vi "Create Registry.vi"(8 "Error In":errorcluster) -> (0 "Error Out":errorcluster)   [LabVIEW 2014]
doc: "This subVI creates a registry for registring and control version numbers."
uses:
  <vilib>/Utility/file.llb/Read From Spreadsheet File (string).vi
panel:
  in  "Enum":enum16{"idle", "create", "cancle"}(ring)
  in  "Cancel Button":bool
  in  "Create":bool
  in  "Project Description":string="GFB HIL project setup. Project no. 7152364"
  in  "Delimiter":string=";"
  in  "Project Name":string="Gullfaks B"
  out "ini file path":path
  # "Create Registry"
  # "This application creates a TDMS file that is used to store version numbers\nof all the executables in the HIL setup.\n\nIf the TDMS file has already been created, avoid running this application. Run Update Registry, instead.\n\nTo run this application, you need a database of the components, saved as a CSV file."
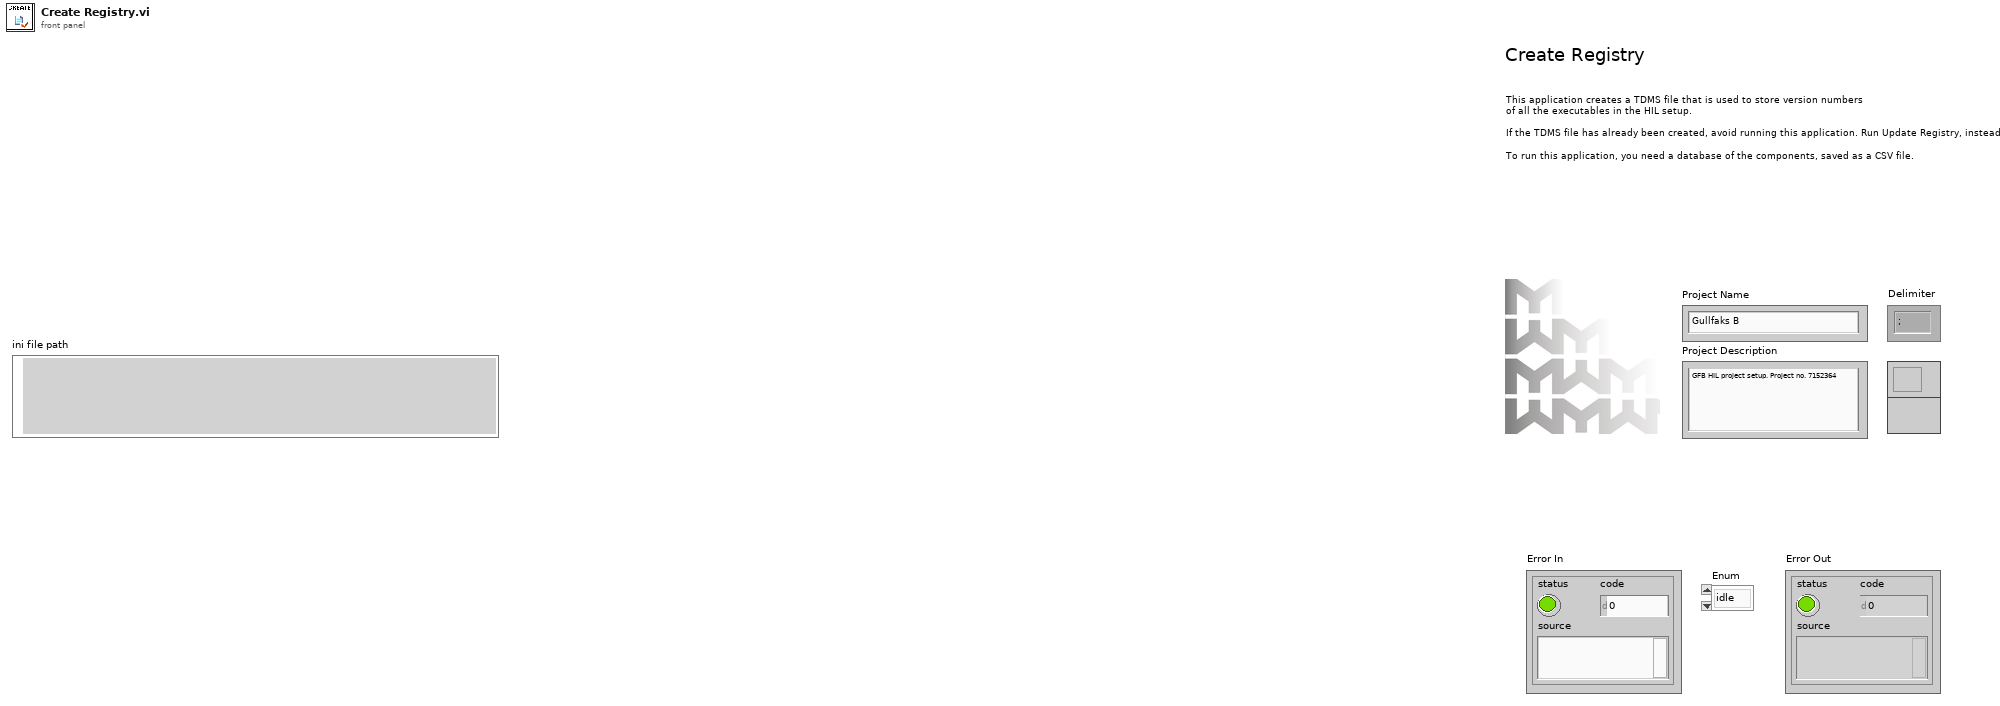
[diagram p1: front panel]
types:
  T1 = cluster{"Folder Path containing version information":path, "File name (including .ini)":path, "Section":string}
  T2 = cluster{"path":path, "This VI":refnum<vi>, "Level of Application":u8}
  T3 = enum16{"open", "open or create", "create or replace", "create", "open (read-only)"}
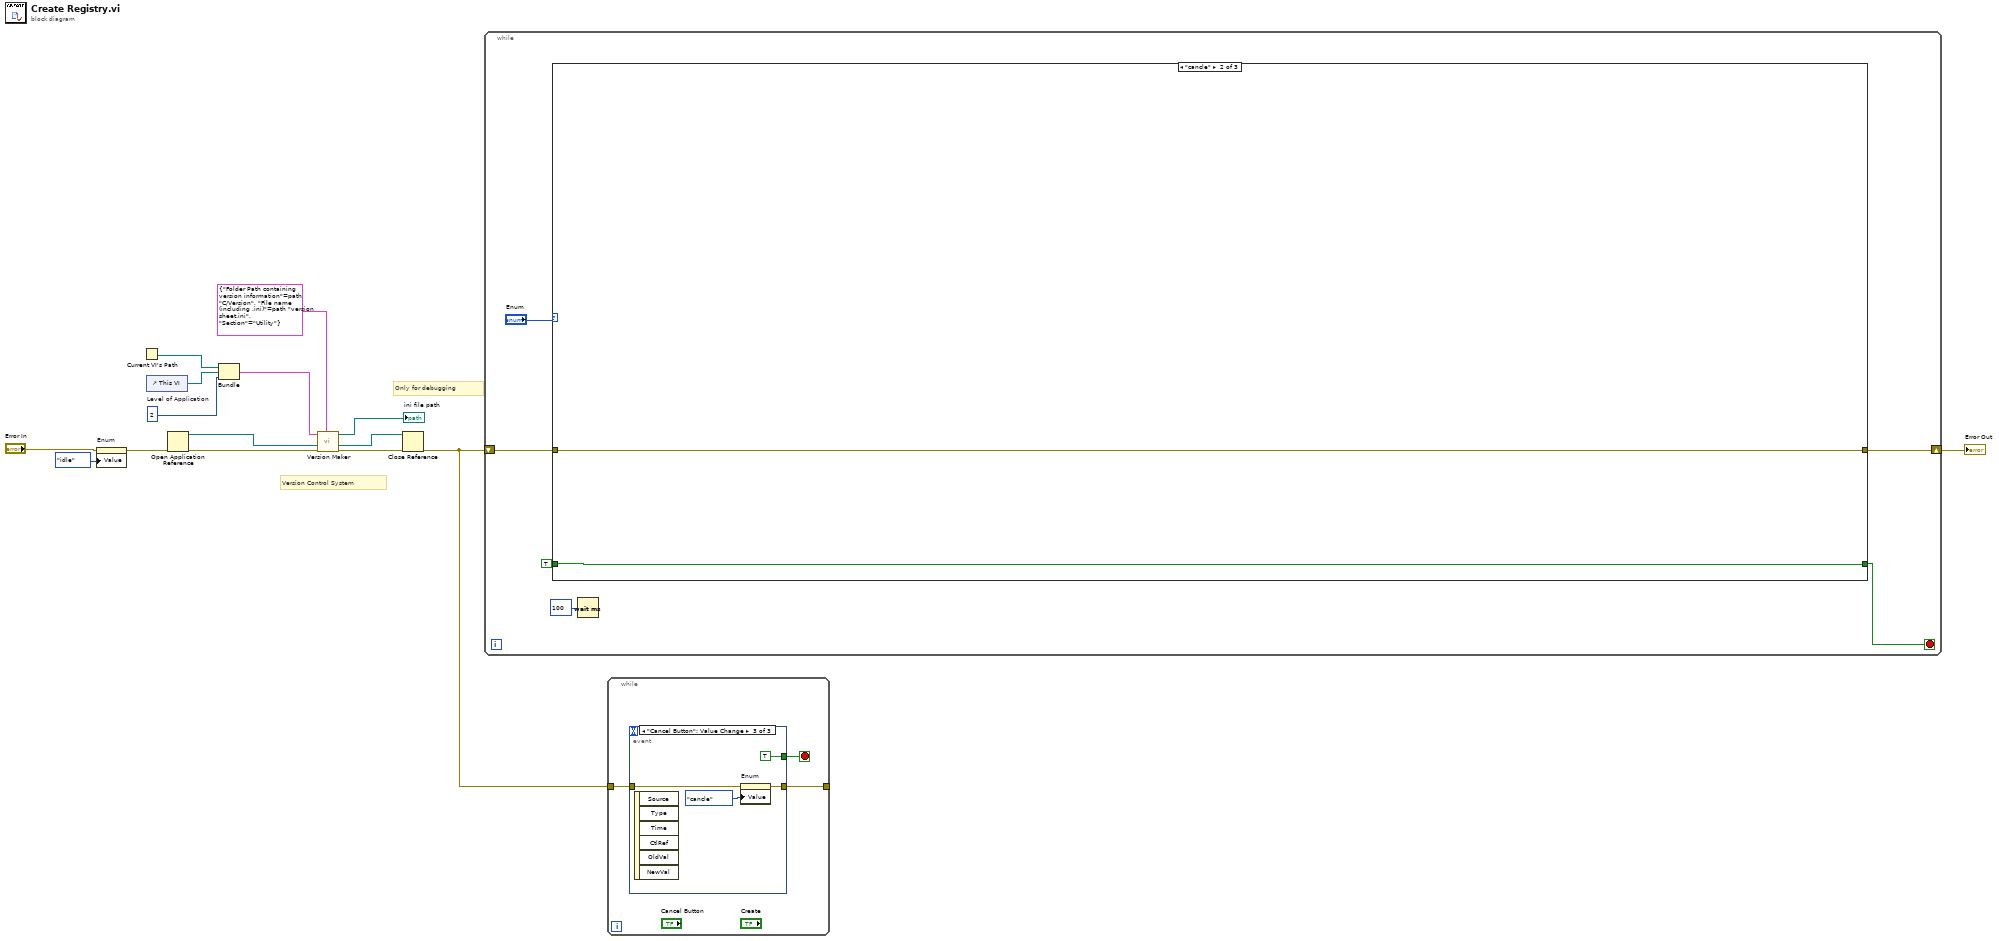
[diagram p0: block diagram]
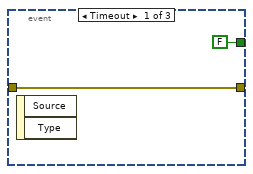
[diagram p2: hidden frame]
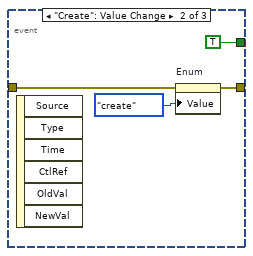
[diagram p3: hidden frame]
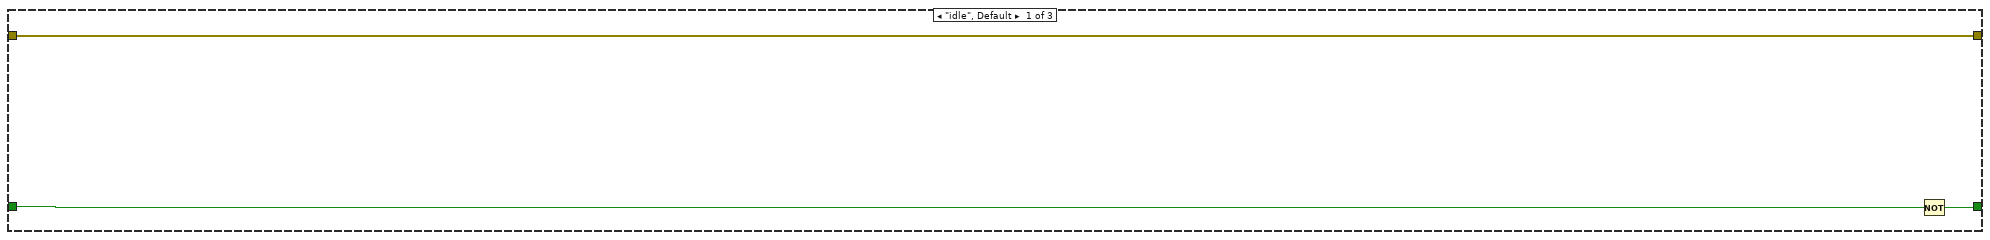
[diagram p4: hidden frame]
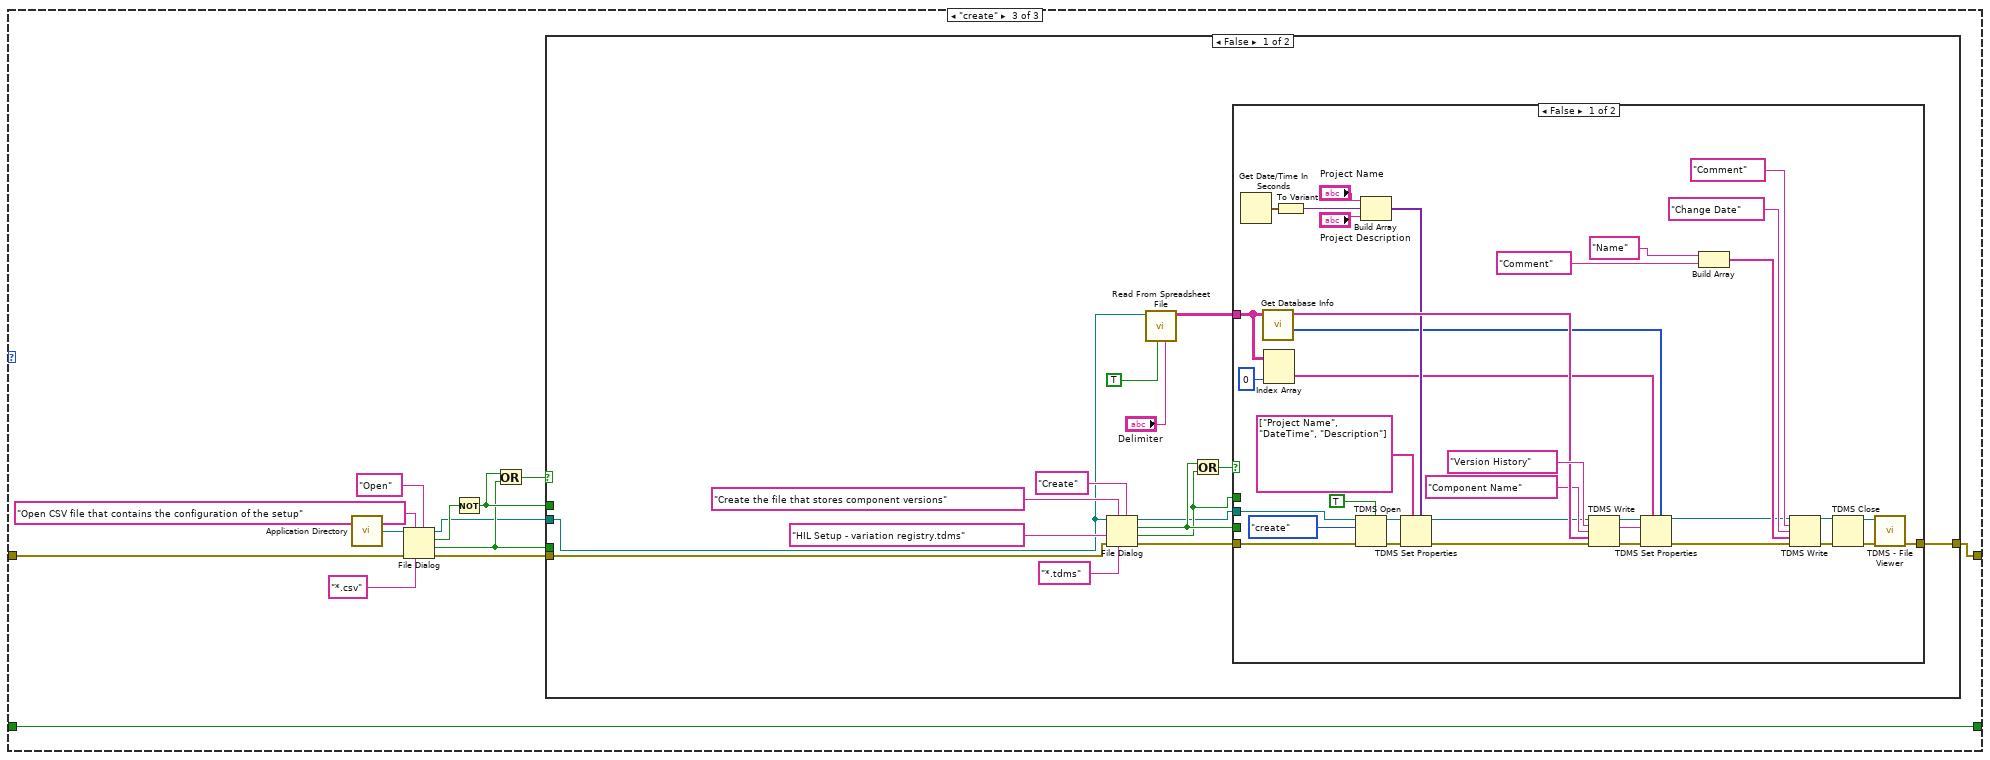
[diagram p5: hidden frame]
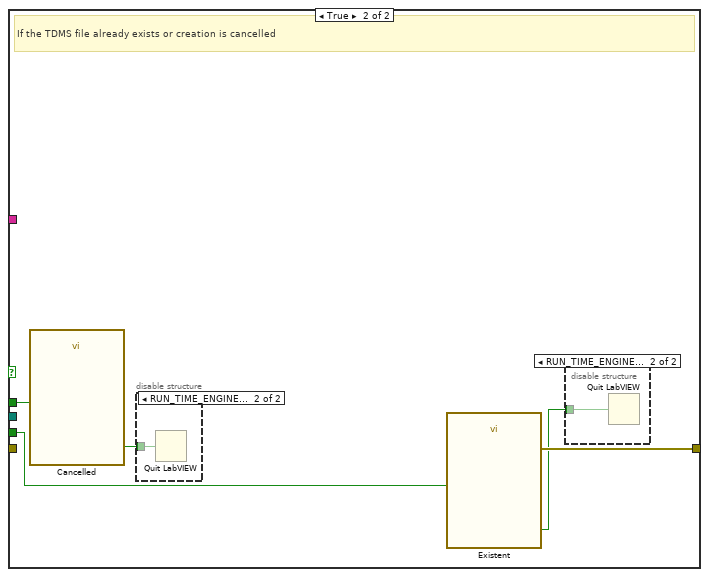
[diagram p6: hidden frame]
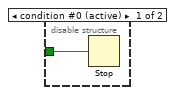
[diagram p7: hidden frame]
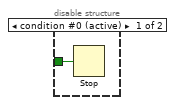
[diagram p8: hidden frame]
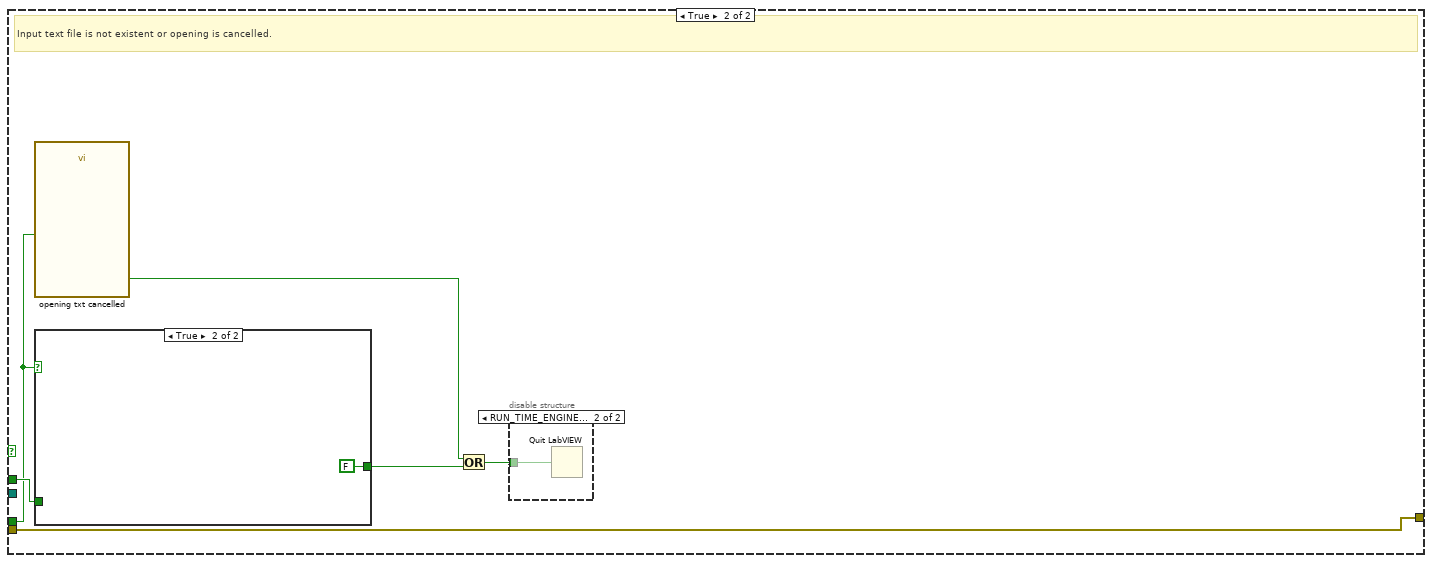
[diagram p9: hidden frame]
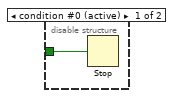
[diagram p10: hidden frame]
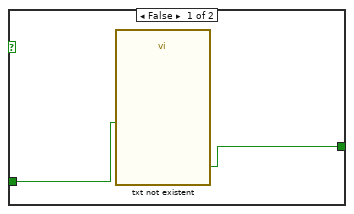
[diagram p11: hidden frame]
diagram:
  w8 = u8 2  # Level of Application
  # "Only for debugging"
  # "Version Control System"
  n1 = property on="Enum" class="Enum (strict)"(error in="Error In", "Value"=enum16{"idle", "create", "cancle"}."idle" ("Enum")) -> (error out=w2:errorcluster)  [unwired: 1 in, 1 out]
  n2 = Current VI's Path() -> (path=w6:path)
  n3 = control-ref of="This VI"() -> (w7:refnum<vi>)
  n4 = Open Application Reference(8:w2) -> (0:w15:errorcluster, 3:w11:refnum<vi>)  [unwired: 3 in]
  n5 = Bundle("path"=w6, "This VI"=w7, "Level of Application"=w8) -> (w9:T2)  [unwired: 1 in]
  n6 = call "Version Maker.vi"("Version Sheet Cluster"=T1 {"Folder Path containing version information"=path "C:/Version", "File name (including .ini)"=path "version sheet.ini", "Section"="Utility"}, "Error In"=w15, "Open Application Reference in"=w11, "VI Information"=w9) -> ("Error Out"=w14:errorcluster, "Open Application Reference out"=w10:refnum<vi>, "Standard Config Path"=→"ini file path":path)  [unwired: 4 in, 1 out]
  n7 = Close Reference(reference=w10, error in (no error)=w14) -> (error out=w1:errorcluster)
  n8 = while {
    shift-right: [w20] -> w5
    shift-left: w1 -> [w21]
    stop <- w18 stop-if-true
    n9 = case shown="\"cancle\"" "Enum" {
      tunnel: w21 -> [w24 w26 w29]
      tunnel: [w24 w26 w28] -> w20
      tunnel: TRUE -> [w22 w25 w27]
      tunnel: [w23 w25 w27] -> w18
      frame "idle", Default {
        n10 = Not(x=w22) -> (.not. x?=w23:bool)
      }
      frame "cancle" {
      }
      frame "create" {
        n11 = call <vilib>:"Application Directory.vi"() -> ("Application Directory"=w30:path)
        n12 = File Dialog(5:"Open" ("button label"), 6:"*.csv" ("default name"), 7:"Open CSV file that contains the configuration of the setup" ("prompt"), 8:w29, 11:w30) -> (0:w32:errorcluster, 1:w33:bool, 2:w36:bool, 3:w31:path)  [unwired: 1 in, 1 out]
        n13 = Not(x=w36) -> (.not. x?=w34:bool)
        n14 = Or(x=w34, y=w33) -> (x .or. y?=w35:bool)
        n15 = case shown="False" w35 {
          tunnel: w34 -> [_ w105]
          tunnel: w33 -> [_ w103]
          tunnel: w32 -> [w46 w104]
          tunnel: [w45 w104] -> w28
          tunnel: w31 -> [w43 _]
          frame False {
            n16 = File Dialog(5:"Create" ("button label"), 6:"*.tdms" ("pattern (all files)"), 7:"Create the file that stores component versions" ("prompt"), 8:w46, 9:"HIL Setup - variation registry.tdms" ("default name"), 11:w43) -> (0:w51:errorcluster, 1:w52:bool, 2:w53:bool, 3:w50:path)  [unwired: 1 out]
            n17 = call-poly <vilib>:"Read From Spreadsheet File.vi"("delimiter (\\t)"="Delimiter", "transpose (no:F)"=TRUE, "file path (dialog if empty)"=w43) -> ("all rows"=w42:string[][])  [unwired: 4 in, 4 out]
            n18 = Or(x=w53, y=w52) -> (x .or. y?=w54:bool)
            n19 = case shown="False" w54 {
              tunnel: w53 -> [_ w95]
              tunnel: w52 -> [_ w94]
              tunnel: w51 -> [w89 _]
              tunnel: w50 -> [w90 _]
              tunnel: [w83 w93] -> w45
              tunnel: w42 -> [w63 _]
              frame False {
                n20 = Get Date/Time In Seconds() -> (seconds since 1Jan1904=w66:timestamp)
                n21 = call "Get Database Info.vi"("2D Array in"=w63) -> ("Array"=w57:u32[], "2D Array in 2"=w75:string[])  [unwired: 9 in]
                n22 = Index Array(array=w63, index (col)=0 ("disabled index (col)")) -> (element=w58:string[])  [unwired: 1 in]
                n23 = To Variant(anything=w66) -> (Variant=w67:variant)
                n24 = TDMS Open(5:TRUE ("create index file? (T)"), 8:w89, 10:T3."create" ("operation (0:open)"), 11:w90) -> (0:w73:errorcluster, 3:w65:refnum<k34>)  [unwired: 3 in]
                n25 = Build Array("Project Name", w67, "Project Description") -> (w68:variant[])
                n26 = TDMS Set Properties(5:w68, 7:string[] ["Project Name", "DateTime", "Description"] ("property names"), 8:w73, 11:w65) -> (0:w72:errorcluster, 3:w71:refnum<k34>)  [unwired: 2 in, 2 out]
                n27 = TDMS Write(0:w71, 5:"Version History" ("group name in (Untitled)"), 7:"Component Name" ("group name in (Untitled)"), 9:w75, 11:w72) -> (4:w60:refnum<k34>, 6:w59:string, 15:w61:errorcluster)  [unwired: 1 in, 1 out]
                n28 = TDMS Set Properties(5:w57, 7:w58, 8:w61, 10:w59, 11:w60) -> (0:w55:errorcluster, 3:w56:refnum<k34>)  [unwired: 1 in, 2 out]
                n29 = Build Array("Name" ("group name in (Untitled)"), "Comment" ("group name in (Untitled)")) -> (w77:string[])
                n30 = TDMS Write(0:w56, 5:"Comment" ("group name in (Untitled)"), 7:"Change Date" ("group name in (Untitled)"), 9:w77, 11:w55) -> (4:w80:refnum<k34>, 15:w79:errorcluster)  [unwired: 1 in, 2 out]
                n31 = TDMS Close(8:w79, 11:w80) -> (0:w85:errorcluster, 3:w84:path)
                n32 = call <vilib>:"TDMS - File Viewer.vi"("error in (no error)"=w85, "file path"=w84) -> ("error out"=w83:errorcluster)  [unwired: 4 in, 1 out]
              }
              frame True {
                # "If the TDMS file already exists or creation is cancelled"
                n33 = call "Cancelled"("Enable"=w94) -> ("OK"=w92:bool)  [unwired: 9 in, 1 out]
                n34 = disable-structure shown="RUN_TIME_ENGINE==True" {
                  disable-tunnel: w92 -> [w98 w99]
                  frame condition #0 (active) {
                    n35 = Stop(stop? (T)=w98) -> ()
                  }
                  frame condition #1 {
                    n36 = Quit LabVIEW(quit? (T)=w99) -> ()
                  }
                }
                n37 = call "Existent"("Enable"=w95) -> ("error out"=w93:errorcluster, "OK"=w91:bool)  [unwired: 9 in]
                n38 = disable-structure shown="RUN_TIME_ENGINE==True" {
                  disable-tunnel: w91 -> [w96 w97]
                  frame condition #0 (active) {
                    n39 = Stop(stop? (T)=w96) -> ()
                  }
                  frame condition #1 {
                    n40 = Quit LabVIEW(quit? (T)=w97) -> ()
                  }
                }
              }
            }
          }
          frame True {
            # "Input text file is not existent or opening is cancelled."
            n41 = call "opening txt cancelled"("Enable"=w103) -> ("OK"=w101:bool)  [unwired: 9 in, 1 out]
            n42 = case shown="True" w103 {
              tunnel: w105 -> [w109 _]
              tunnel: [w108 FALSE ("OK")] -> w102
              frame False {
                n43 = call "txt not existent"("Enable"=w109) -> ("OK"=w108:bool)  [unwired: 9 in, 1 out]
              }
              frame True {
              }
            }
            n44 = Or(x=w101, y=w102) -> (x .or. y?=w100:bool)
            n45 = disable-structure shown="RUN_TIME_ENGINE==True" {
              disable-tunnel: w100 -> [w106 w107]
              frame condition #0 (active) {
                n46 = Stop(stop? (T)=w106) -> ()
              }
              frame condition #1 {
                n47 = Quit LabVIEW(quit? (T)=w107) -> ()
              }
            }
          }
        }
      }
    }
    n48 = Wait (ms)(milliseconds to wait=u32 100) -> ()  [unwired: 1 out]
  }
  "Error Out" <- w5
  n49 = while {
    tunnel: w1 -> [w113]
    tunnel: [w112] -> _
    stop <- w111 stop-if-true
    n50 = event shown="[2] \"Cancel Button\": Value Change" {
      selector: _ -> [_ _ _]
      dyn-events: _ -> [_ _ _]
      timeout: _ -> [_ _ _]
      tunnel: w113 -> [w114 w118 w122]
      tunnel: [w114 w117 w121] -> w112
      tunnel: [FALSE TRUE TRUE] -> w111
      event Timeout {
        n51 = event-data() -> ()  [unwired: 1 in, 2 out]
      }
      event "Create": Value Change {
        n52 = event-data() -> ()  [unwired: 1 in, 6 out]
        n53 = property on="Enum" class="Enum (strict)"(error in=w118, "Value"=enum16{"idle", "create", "cancle"}."create" ("Enum")) -> (error out=w117:errorcluster)  [unwired: 1 in, 1 out]
      }
      event "Cancel Button": Value Change {
        n54 = event-data() -> ()  [unwired: 1 in, 6 out]
        n55 = property on="Enum" class="Enum (strict)"(error in=w122, "Value"=enum16{"idle", "create", "cancle"}."cancle" ("Enum")) -> (error out=w121:errorcluster)  [unwired: 1 in, 1 out]
      }
    }
  }
